vi "Read DVR_voltage.vi"(8 "error in (no error)":errorcluster, 11 "DAQ Voltage in":refnum<class "DAQ Voltage.lvclass">) -> (0 "error out":errorcluster, 2 "DVR_voltage":refnum<data-value>, 3 "DAQ Voltage out":refnum<class "DAQ Voltage.lvclass">)   [LabVIEW 2025, in "DAQ Voltage.lvlib" / "DAQ Voltage.lvclass"]
uses:
  DAQ Voltage.lvclass
  DAQ Voltage.lvclass/DAQ Voltage.ctl
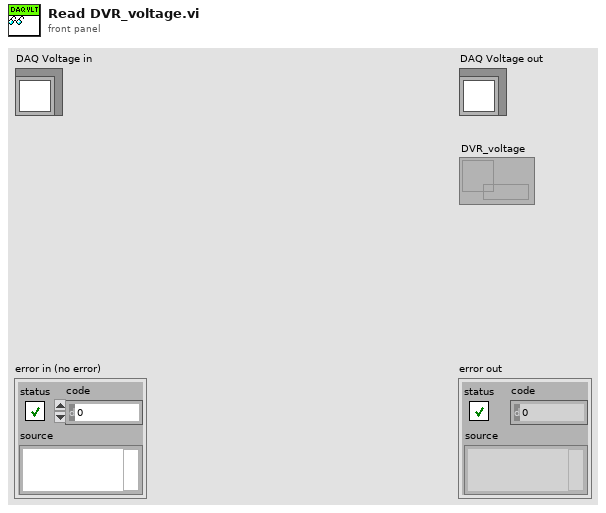
[diagram p1: front panel]
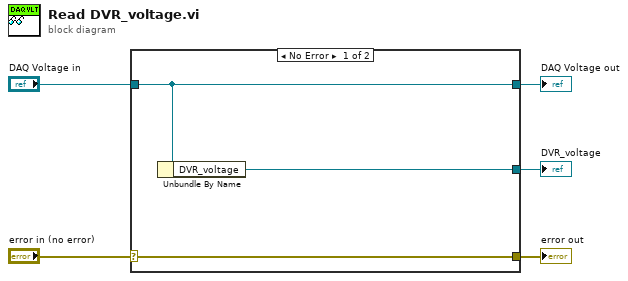
[diagram p0: block diagram]
diagram:
  n1 = case shown="No Error" "error in (no error)" {
    selector: "error in (no error)" -> [w8 w9]
    tunnel: [w8 w9] -> w4
    tunnel: [w7 w10] -> w2
    tunnel: "DAQ Voltage in" -> [w7 w10]
    tunnel: [w6 _] -> w1
    frame No Error {
      n2 = Unbundle By Name(w7) -> ("DVR_voltage"=w6:refnum<data-value>)
    }
    frame Error {
    }
  }
  "error out" <- w4
  "DAQ Voltage out" <- w2
  "DVR_voltage" <- w1
